vi "EXP-2.vi"() -> ()   [LabVIEW 2013]
panel:
  out "output":dbl
  in  "constant":i32
  in  "Numeric 2":dbl
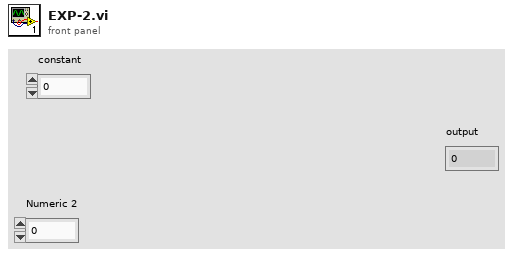
[diagram p1: front panel]
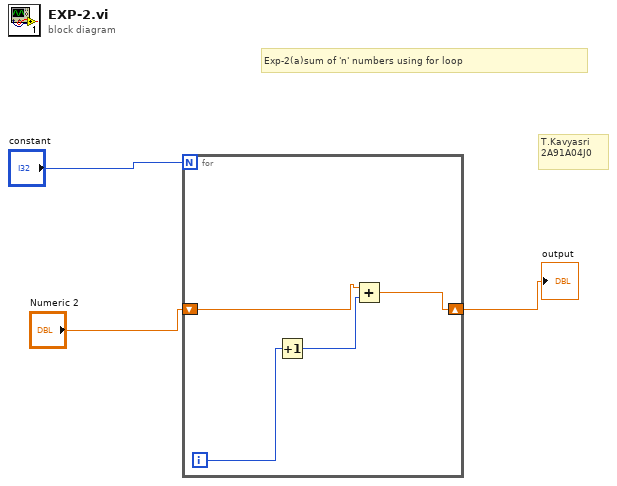
[diagram p0: block diagram]
diagram:
  # "T.Kavyasri\n2A91A04J0"
  # "Exp-2(a)sum of 'n' numbers using for loop"
  n1 = for {
    N: "constant" -> [_]
    shift-right: [w4] -> w1
    shift-left: "Numeric 2" -> [w5]
    i -> [w7]
    n2 = Increment(x=w7) -> (x+1=w6:i32)
    n3 = Add(x=w5, y=w6) -> (x+y=w4:dbl)
  }
  "output" <- w1
